vi "SourceCloseSynchronization.vi"(0 "error in (no error)":errorcluster, 1 "Queue Reference in":refnum<notifier>[](array[refnum]), 2 "Notifiers in":refnum<notifier>[](array[refnum]), 4 "Queue in":refnum<queue>) -> (3 "error out (no error)":errorcluster caption="error out")   [LabVIEW 2009]
uses:
  Controls/SourceCommand.ctl
  Controls/SourceStatus.ctl
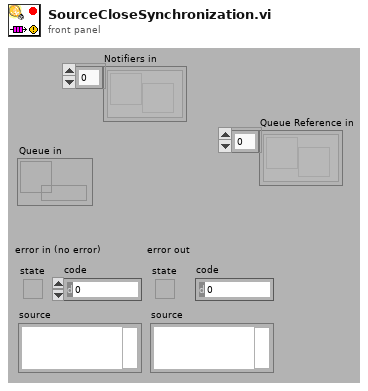
[diagram p1: front panel]
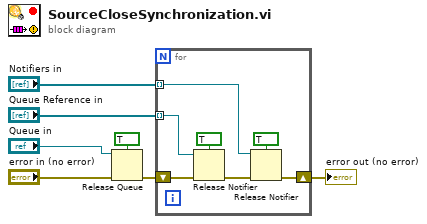
[diagram p0: block diagram]
diagram:
  n1 = Release Queue(queue="Queue in", force destroy? (F)=TRUE ("forcer la destruction ? (F)"), error in (no error)="error in (no error)") -> (error out=w6:errorcluster)  [unwired: 2 out]
  n2 = for {
    tunnel: "Notifiers in" -> [w13] mode=indexing
    shift-right: [w14] -> w7
    shift-left: w6 -> [w10]
    tunnel: "Queue Reference in" -> [w8] mode=indexing
    n3 = Release Notifier(notifier=w8, force destroy? (F)=TRUE ("forcer la destruction ? (F)"), error in (no error)=w10) -> (error out=w9:errorcluster)  [unwired: 2 out]
    n4 = Release Notifier(notifier=w13, force destroy? (F)=TRUE ("forcer la destruction ? (F)"), error in (no error)=w9) -> (error out=w14:errorcluster)  [unwired: 2 out]
  }
  "error out (no error)" <- w7
